vi "Ocean Optics 2000 4000 Spectrometer Setup.vi"() -> ()   [LabVIEW 2021]
doc: "Demontrates the integration time, trigger and strobe setup."
uses:
  <instrlib>/Ocean Optics 2000 4000/Ocean Optics 2000 4000.lvlib
panel:
  in  "Continuous Strobe Divisor (4800)":u16=4800
  in  "Continuous Strobe Base Clock Divisor (48000)":u16=48000
  in  "Single Strobe Low Transitional Delay Counter (5)":u16=5
  in  "Single Strobe High Transitional Delay Counter (1)":u16=1
  in  "Enable Strobe (Disabled)":bool
  in  "Hardware Trigger Delay (0 s)":u16
  in  "Trigger Type (0:Normal)":u8(ring) items=["Normal", "Software Trigger Mode", "External Sync Trigger Mode", "External Hardware Trigger Mode"]
  in  "Integration Time (6000us)":u32=6000
  in  "VISA resource name":refnum<visa-resource-name>
  # "(c) 2009-2016 National Instruments.  ALL RIGHTS RESERVED."
  # "Strobe Control"
  # "Trigger Control"
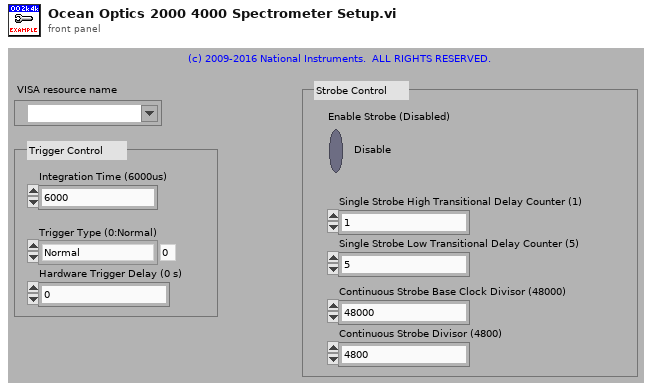
[diagram p1: front panel]
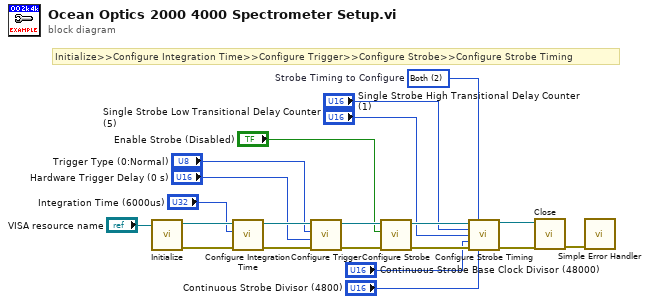
[diagram p0: block diagram]
diagram:
  w4 = u16 2 items=["Single Strobe", "Continuous Strobe", "Both"]  # Strobe Timing to Configure
  # "Initialize>>Configure Integration Time>>Configure Trigger>>Configure Strobe>>Configure Strobe Timing"
  n1 = call <instrlib>:"Initialize.vi"("VISA resource name"="VISA resource name") -> ("error out"=w19:errorcluster, "VISA resource name out"=w20:refnum<visa-resource-name>)  [unwired: 2 in, 7 out]
  n2 = call <instrlib>:"Configure Integration Time.vi"("error in (no error)"=w19, "Integration Time (6000)"="Integration Time (6000us)", "VISA resource name"=w20) -> ("error out"=w17:errorcluster, "VISA resource name out"=w18:refnum<visa-resource-name>)  [unwired: 7 out]
  n3 = call <instrlib>:"Configure Trigger.vi"("error in (no error)"=w17, "Hardware Trigger Delay (0 s)"="Hardware Trigger Delay (0 s)", "Trigger Type (0:Normal)"="Trigger Type (0:Normal)", "VISA resource name"=w18) -> ("error out"=w15:errorcluster, "VISA resource name out"=w16:refnum<visa-resource-name>)  [unwired: 6 out]
  n4 = call <instrlib>:"Configure Strobe.vi"("error in (no error)"=w15, "Enable Strobe (Disabled)"="Enable Strobe (Disabled)", "VISA resource name"=w16) -> ("error out"=w13:errorcluster, "VISA resource name out"=w14:refnum<visa-resource-name>)  [unwired: 7 out]
  n5 = call <instrlib>:"Configure Strobe Timing.vi"("VISA resource name"=w14, "Strobe Timing to Configure (2:Both)"=w4, "Single Strobe High Transitional Delay Counter (1)"="Single Strobe High Transitional Delay Counter (1)", "Single Strobe Low Transitional Delay Counter (5)"="Single Strobe Low Transitional Delay Counter (5)", "Continuous Strobe Base Clock Divisor (48000)"="Continuous Strobe Base Clock Divisor (48000)", "error in (no error)"=w13, "Continuous Strobe Divisor (4800)"="Continuous Strobe Divisor (4800)") -> ("VISA resource name out"=w3:refnum<visa-resource-name>, "error out"=w2:errorcluster)  [unwired: 1 in, 6 out]
  n6 = call <instrlib>:"Close.vi"("error in (no error)"=w2, "VISA resource name"=w3) -> ("error out"=w1:errorcluster)  [unwired: 9 out]
  n7 = call <vilib>:"Simple Error Handler.vi"("error in (no error)"=w1) -> ()  [unwired: 1 in, 8 out]
